vi "RemoveDelay.vi"(3 "Delay, ns":u32=6000, 4 "Time High":u32, 5 "Time Low":u32) -> (1 "Time High New":u32, 2 "Time Low New":u32)   [LabVIEW 2009]
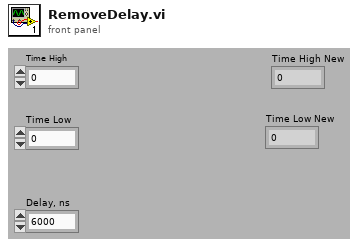
[diagram p1: front panel]
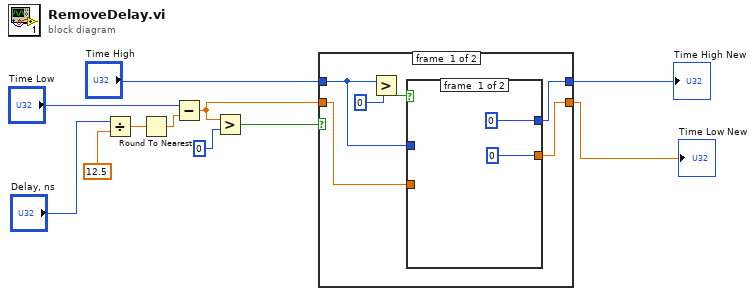
[diagram p0: block diagram]
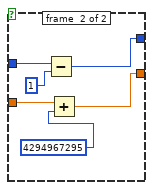
[diagram p2: hidden frame]
diagram:
  n1 = Divide(x="Delay, ns", y=12.5) -> (x/y=w2:dbl)
  n2 = Round To Nearest(number=w2) -> (nearest integer value=w1:dbl)
  n3 = Subtract(x="Time Low", y=w1) -> (x-y=w8:dbl)
  n4 = Greater?(x=w8, y=0) -> (0:w9:bool)
  n5 = case shown="False" w9 {
    tunnel: w8 -> [w12 w26]
    tunnel: "Time High" -> [w13 w27]
    tunnel: [w15 w27] -> w6
    tunnel: [w14 w26] -> w5
    frame #0 {
      n6 = Greater?(x=w13, y=0) -> (0:w16:bool)
      n7 = case shown="True" w16 {
        tunnel: [0 w20] -> w15
        tunnel: [0 w23] -> w14
        tunnel: w13 -> [_ w22]
        tunnel: w12 -> [_ w25]
        frame #0 {
        }
        frame #1 {
          n8 = Subtract(x=w22, y=1) -> (x-y=w20:u32)
          n9 = Add(x=w25, y=u32 4294967295) -> (x+y=w23:dbl)
        }
      }
    }
    frame #1 {
    }
  }
  "Time High New" <- w6
  "Time Low New" <- w5
